vi "SortTC_Display.vi"(11 "TCData":T1) -> (3 "TCsDisplay":T2={"TC0_LP1_Hi"=25.446637506096643, "TC1_LP1_MidHi"=-67954.67080824148, "TC2_LP1_Mid"=-67954.0860092046, "TC3_LP1_LoMid"=-68014.21654976695, "TC4_LP1_Lo"=-68013.6313297234, "TC5_LP2_Hi"=-68014.21654976695, "TC6_LP2_MidHi"=-68058.43020070596, "TC7_LP2_Mid"=-68059.01573745323, "TC8_LP2_LoMid"=-67937.01745222262, "TC9_LP2_Lo"=-67937.60213056742, "TC10_HVAC_Cond_In"=-67937.01745222262, "TC11_HVAC_Cond_Out"=-68021.98391844248, "TC12_Gen_Exhaust"=-68021.39864348577, "TC13_Tamb_Interior"=-68021.39864348577} caption="Thermocouples" {"TC13_Tamb_Interior" format="%#.1f"; "TC12_Gen_Exhaust" format="%#.1f"; "TC11_HVAC_Cond_Out" format="%#.1f"; "TC10_HVAC_Cond_In" format="%#.1f"; "TC9_LP2_Lo" format="%#.1f"; "TC8_LP2_LoMid" format="%#.1f"; "TC7_LP2_Mid" format="%#.1f"; "TC6_LP2_MidHi" format="%#.1f"; "TC5_LP2_Hi" format="%#.1f"; "TC4_LP1_Lo" format="%#.1f"; "TC3_LP1_LoMid" format="%#.1f"; "TC2_LP1_Mid" format="%#.1f"; "TC1_LP1_MidHi" format="%#.1f"; "TC0_LP1_Hi" format="%#.1f"})   [LabVIEW 2018]
uses:
  Controls/Clusts/TC_Display_Clust.ctl
  HDF5/TC_Data_Structure.ctl
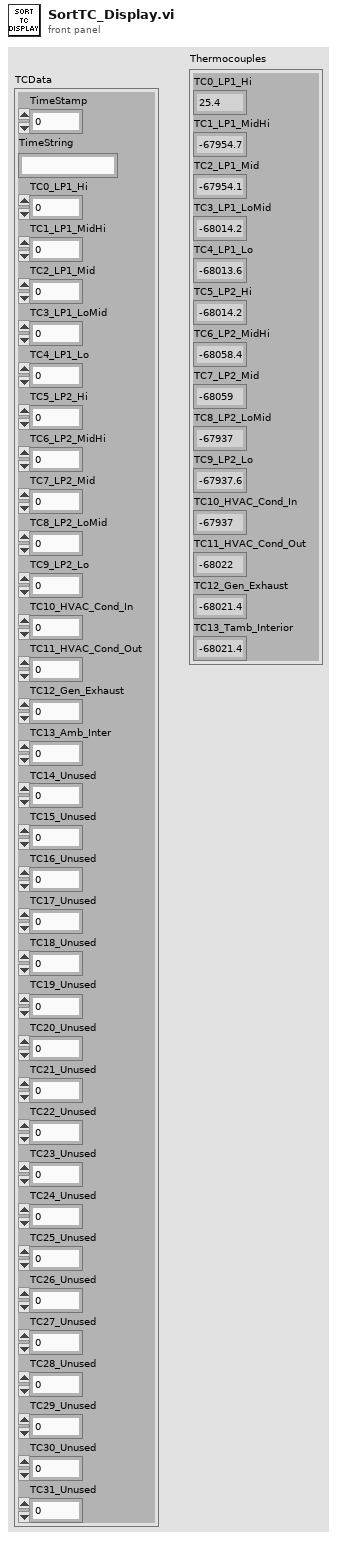
[diagram p1: front panel]
types:
  T1 = typedef "TC_Data_Structure.ctl" = cluster{"TimeStamp":dbl, "TimeString":string, "TC0_LP1_Hi":dbl, "TC1_LP1_MidHi":dbl, "TC2_LP1_Mid":dbl, "TC3_LP1_LoMid":dbl, "TC4_LP1_Lo":dbl, "TC5_LP2_Hi":dbl, "TC6_LP2_MidHi":dbl, "TC7_LP2_Mid":dbl, "TC8_LP2_LoMid":dbl, "TC9_LP2_Lo":dbl, "TC10_HVAC_Cond_In":dbl, "TC11_HVAC_Cond_Out":dbl, "TC12_Gen_Exhaust":dbl, "TC13_Amb_Inter":dbl, "TC14_Unused":dbl, "TC15_Unused":dbl, "TC16_Unused":dbl, "TC17_Unused":dbl, "TC18_Unused":dbl, "TC19_Unused":dbl, "TC20_Unused":dbl, "TC21_Unused":dbl, "TC22_Unused":dbl, "TC23_Unused":dbl, "TC24_Unused":dbl, "TC25_Unused":dbl, "TC26_Unused":dbl, "TC27_Unused":dbl, "TC28_Unused":dbl, "TC29_Unused":dbl, "TC30_Unused":dbl, "TC31_Unused":dbl}
  T2 = typedef "TC_Display_Clust.ctl" = cluster{"TC0_LP1_Hi":dbl, "TC1_LP1_MidHi":dbl, "TC2_LP1_Mid":dbl, "TC3_LP1_LoMid":dbl, "TC4_LP1_Lo":dbl, "TC5_LP2_Hi":dbl, "TC6_LP2_MidHi":dbl, "TC7_LP2_Mid":dbl, "TC8_LP2_LoMid":dbl, "TC9_LP2_Lo":dbl, "TC10_HVAC_Cond_In":dbl, "TC11_HVAC_Cond_Out":dbl, "TC12_Gen_Exhaust":dbl, "TC13_Tamb_Interior":dbl}
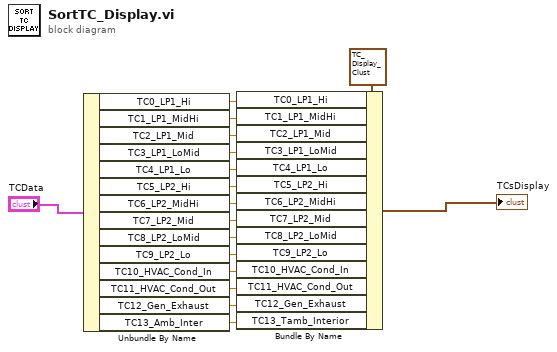
[diagram p0: block diagram]
diagram:
  n1 = Unbundle By Name("TCData") -> ("TC0_LP1_Hi"=w3:dbl, "TC1_LP1_MidHi"=w4:dbl, "TC2_LP1_Mid"=w5:dbl, "TC3_LP1_LoMid"=w6:dbl, "TC4_LP1_Lo"=w7:dbl, "TC5_LP2_Hi"=w8:dbl, "TC6_LP2_MidHi"=w9:dbl, "TC7_LP2_Mid"=w10:dbl, "TC8_LP2_LoMid"=w11:dbl, "TC9_LP2_Lo"=w12:dbl, "TC10_HVAC_Cond_In"=w13:dbl, "TC11_HVAC_Cond_Out"=w14:dbl, "TC12_Gen_Exhaust"=w15:dbl, "TC13_Amb_Inter"=w1:dbl)
  n2 = Bundle By Name(cluster=T2 {"TC0_LP1_Hi"=25.446637506096643, "TC1_LP1_MidHi"=-67954.67080824148, "TC2_LP1_Mid"=-67954.0860092046, "TC3_LP1_LoMid"=-68014.21654976695, "TC4_LP1_Lo"=-68013.6313297234, "TC5_LP2_Hi"=-68014.21654976695, "TC6_LP2_MidHi"=-68058.43020070596, "TC7_LP2_Mid"=-68059.01573745323, "TC8_LP2_LoMid"=-67937.01745222262, "TC9_LP2_Lo"=-67937.60213056742, "TC10_HVAC_Cond_In"=-67937.01745222262, "TC11_HVAC_Cond_Out"=-68021.98391844248, "TC12_Gen_Exhaust"=-68021.39864348577, "TC13_Tamb_Interior"=-68021.39864348577} ("TCsDisplay"), "TC0_LP1_Hi"=w3, "TC1_LP1_MidHi"=w4, "TC2_LP1_Mid"=w5, "TC3_LP1_LoMid"=w6, "TC4_LP1_Lo"=w7, "TC5_LP2_Hi"=w8, "TC6_LP2_MidHi"=w9, "TC7_LP2_Mid"=w10, "TC8_LP2_LoMid"=w11, "TC9_LP2_Lo"=w12, "TC10_HVAC_Cond_In"=w13, "TC11_HVAC_Cond_Out"=w14, "TC12_Gen_Exhaust"=w15, "TC13_Tamb_Interior"=w1) -> (→"TCsDisplay":T2)
